vi "Clusterwitharrayenum.vi"(1 "Cluster In":T2) -> (0 "Cluster Out":T1)   [LabVIEW 2013]
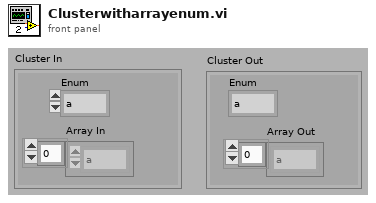
[diagram p1: front panel]
types:
  T1 = cluster{"Array Out":enum16{"a", "b", "c", "d"}[], "Enum":enum16{"a", "b", "c", "d"}}
  T2 = cluster{"Array In":enum16{"a", "b", "c", "d"}[], "Enum":enum16{"a", "b", "c", "d"}}
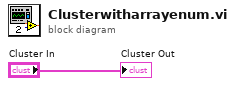
[diagram p0: block diagram]
diagram:
  "Cluster Out" <- "Cluster In"
